vi "Locate Marker.vi"(8 "Marker Image":T2=refnum, 11 "IO Cluster In":T3={"Error"={"status"=FALSE, "code"=0, "source"=""}, "Encoder Calibration Values"=[22, 216], "Update Calibration"=FALSE, "JPEG Resolutions"=3, "Raw Resolutions"=1, "Image Mode"=enum."RAW Gray Scale", "FPGA Ref"=refnum} {"JPEG Resolutions" items=["160x128"=3, "320x240"=5, "640x480"=7]; "Raw Resolutions" items=["80x60"=1, "160x120"=3, "128x128"=9, "128x96"=11]}) -> (3 "Marker Calibration Cluster":T1, 5 "Found Match":bool)   [LabVIEW 2018]
uses:
  QNET MS IO Cluster.ctl
  <vilib>/vision/Image Controls.llb/IMAQ Image.ctl
  <vilib>/vision/NI_Vision_Development_Module.lvlib
panel:
  out "error out":errorcluster
  out "Reference Image":T2(plugin-control)
  out "Acquired Image":T2(plugin-control)
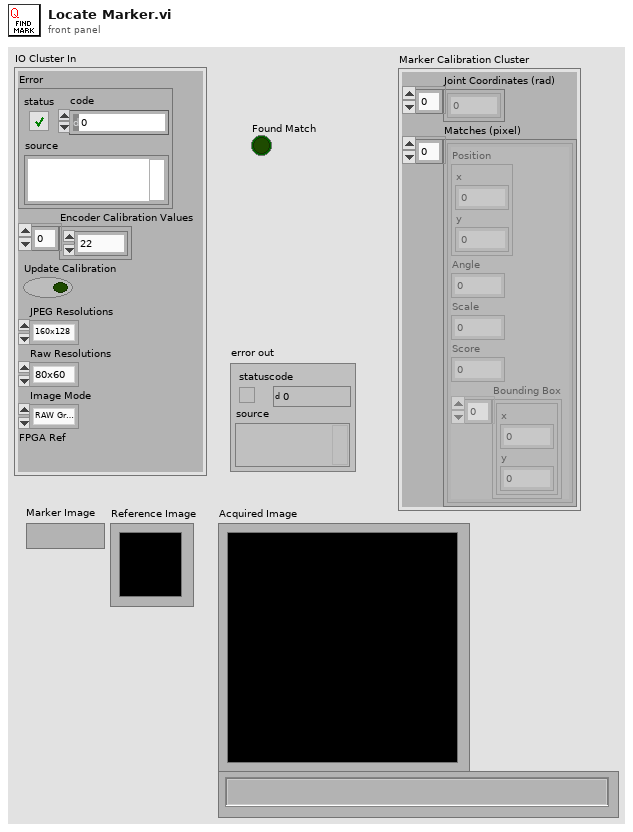
[diagram p1: front panel]
types:
  T1 = cluster{"Joint Coordinates (rad)":dbl[], "Matches (pixel)":cluster{"Position":cluster{"x":sgl, "y":sgl}, "Angle":sgl, "Scale":sgl, "Score":sgl, "Bounding Box":cluster{"x":sgl, "y":sgl}[]}[]}
  T2 = typedef "IMAQ Image.ctl" = refnum<image>
  T3 = typedef "QNET MS IO Cluster.ctl" = cluster{"Error":errorcluster, "Encoder Calibration Values":i32[], "Update Calibration":bool, "JPEG Resolutions":u16, "Raw Resolutions":u16, "Image Mode":enum16{"RAW RGB", "RAW Gray Scale", "JPEG"}, "FPGA Ref":refnum<k20>}
  T4 = typedef "Image Type" = u32
  T5 = cluster{"Algorithm":i32, "Number of Matches Requested":i32, "Minimum Match Score":sgl, "SubPixel Accuracy":bool, "Rotation Angle Ranges":cluster{"Start":sgl, "End":sgl}[], "Show Search Area":bool, "Show Result":bool}
  T6 = cluster{"Position":cluster{"x":sgl, "y":sgl}, "Angle":sgl, "Scale":sgl, "Score":sgl, "Bounding Box":cluster{"x":sgl, "y":sgl}[]}[]
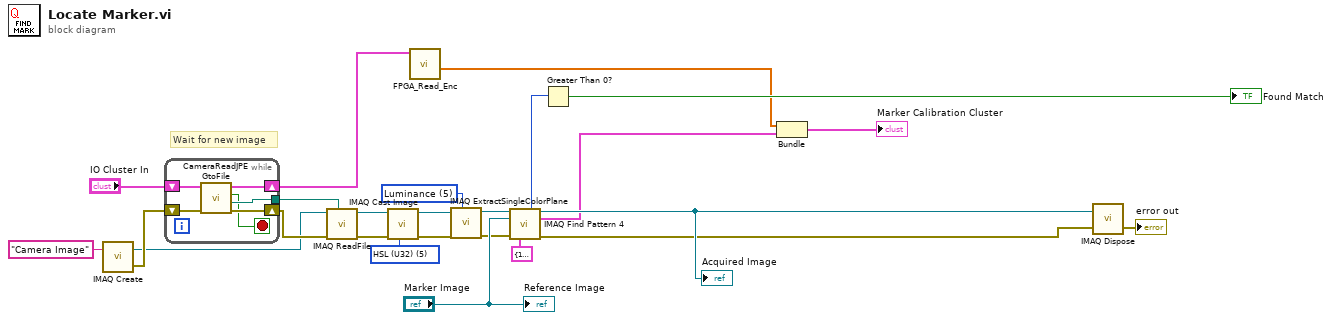
[diagram p0: block diagram]
diagram:
  w9 = 5 items=["Red", "Green", "Blue", "Hue", "Saturation", "Luminance", "Value", "Intensity"] ("Color Plane")
  w10 = T4 5 items=["Grayscale (U8)", "Grayscale (I16)", "Grayscale (SGL)", "Complex (CSG)", "RGB (U32)", "HSL (U32)", "RGB (U64)", "Grayscale (U16)"] ("Image Type")
  # "Wait for new image"
  n1 = call "IMAQ Create"("Image Name"="Camera Image") -> ("New Image"=w18:T2, "error out"=w21:errorcluster)  [unwired: 4 in]
  n2 = while {
    tunnel: [w31] -> w25
    shift-right: [w27] -> w4
    shift-left: "IO Cluster In" -> [w29]
    shift-right: [w30] -> w24
    shift-left: w21 -> [w28]
    stop <- w26 stop-if-true
    n3 = call "CameraReadJPEGtoFile.vi"("error in"=w28, "IO Cluster In"=w29) -> ("Error Out"=w30:errorcluster, "Image File"=w31:path, "New Image Data"=w26:bool, "IO Cluster Out"=w27:T3)  [unwired: 6 in]
  }
  n4 = call "IMAQ ReadFile"("File Path"=w25, "error in (no error)"=w24, "Image"=w18) -> ("error out"=w6:errorcluster, "Image Out"=w5:T2)  [unwired: 4 in, 3 out]
  n5 = call "IMAQ Cast Image"("Image Type"=w10, "error in (no error)"=w6, "Image Src"=w5) -> ("error out"=w7:errorcluster, "Image Dst Out"=w8:T2)  [unwired: 7 in]
  n6 = call "FPGA_Read_Enc.vi"("IO Cluster In"=w4) -> ("Joint Coordinates (rad)"=w3:dbl[])  [unwired: 8 in, 2 out]
  n7 = call "IMAQ ExtractSingleColorPlane"("Color Plane"=w9, "error in (no error)"=w7, "Image Src"=w8) -> ("error out"=w11:errorcluster, "Image Dst Out"=w12:T2)  [unwired: 7 in]
  n8 = call "IMAQ Find Pattern 4"("Image"=w12, "Template"="Marker Image", "error in"=w11, "Settings"=T5 {"Algorithm"=1, "Number of Matches Requested"=1, "Minimum Match Score"=650.0, "SubPixel Accuracy"=TRUE, "Rotation Angle Ranges"=[{"Start"=0.0, "End"=360.0}], "Show Search Area"=TRUE, "Show Result"=TRUE}) -> ("Number of Matches"=w13:i32, "Image Out"=w20:T2, "Matches (pixel)"=w2:T6, "error out"=w19:errorcluster)  [unwired: 5 in, 3 out]
  "Acquired Image" <- w20
  n9 = Greater Than 0?(x=w13) -> (x > 0?=→"Found Match":bool)
  n10 = Bundle("Joint Coordinates (rad)"=w3, "Matches (pixel)"=w2) -> (→"Marker Calibration Cluster":T1)  [unwired: 1 in]
  n11 = call "IMAQ Dispose"("Image"=w20, "error in (no error)"=w19) -> ("error out"=→"error out":errorcluster)  [unwired: 4 in]
  "Reference Image" <- "Marker Image"
